vi "fpga_test.vi"() -> ()   [LabVIEW 2012]
uses:
  <vilib>/Utility/file.llb/Read From Spreadsheet File (I64).vi
panel:
  out "Array":i16[](array[numeric])
  out "unsigned 8bit integer":u8
  out "decimal integer string":string
  out "all rows 2":i64[][](array[numeric])
  out "all rows":i64[][](array[numeric])
  out "Starting address":u32
  out "State":enum16{"Wait for Command", "Read Buffer"}(ring)
  out "Is trigger?":bool
  out "count":u32
  out "Data":i16
  out "Timestamp":u64
  out "Channel":u8
  out "Trigger index":u32
  in  "Record Size only data":u32=95
  in  "circular buffer length":u32=1000
  in  "location":i16(ring) items=["Purdue", "NIKHEF", "Zurich", "???"]
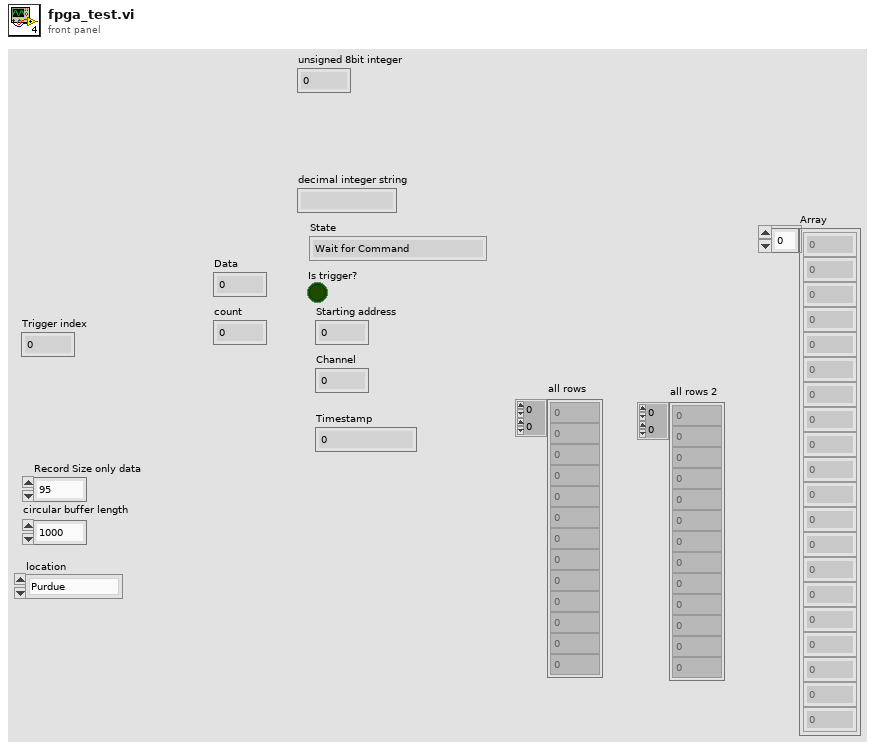
[diagram p1: front panel]
types:
  T1 = enum16{"open", "replace", "create", "open or create", "replace or create", "replace or create with confirmation"}
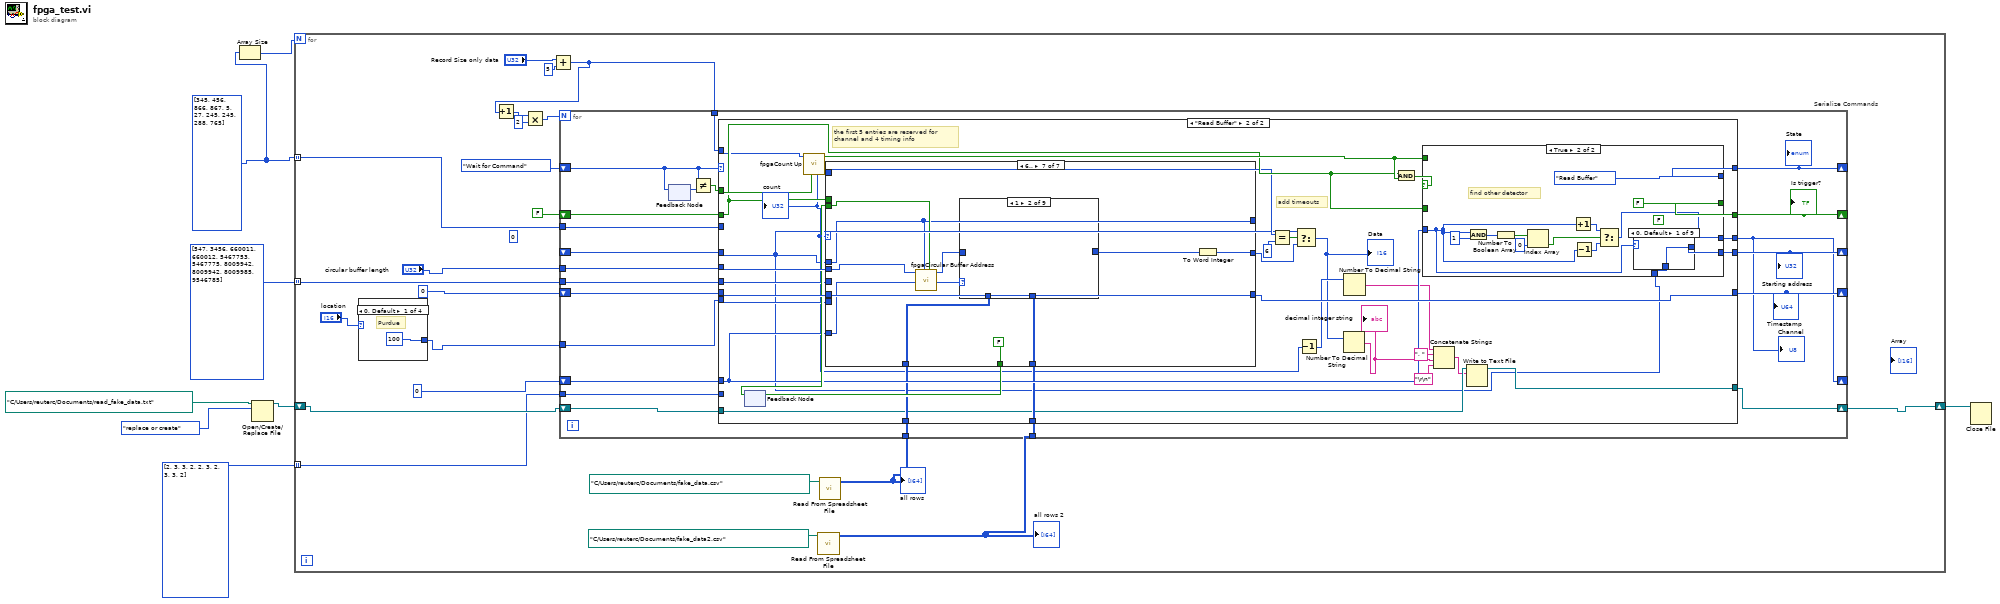
[diagram p0: block diagram]
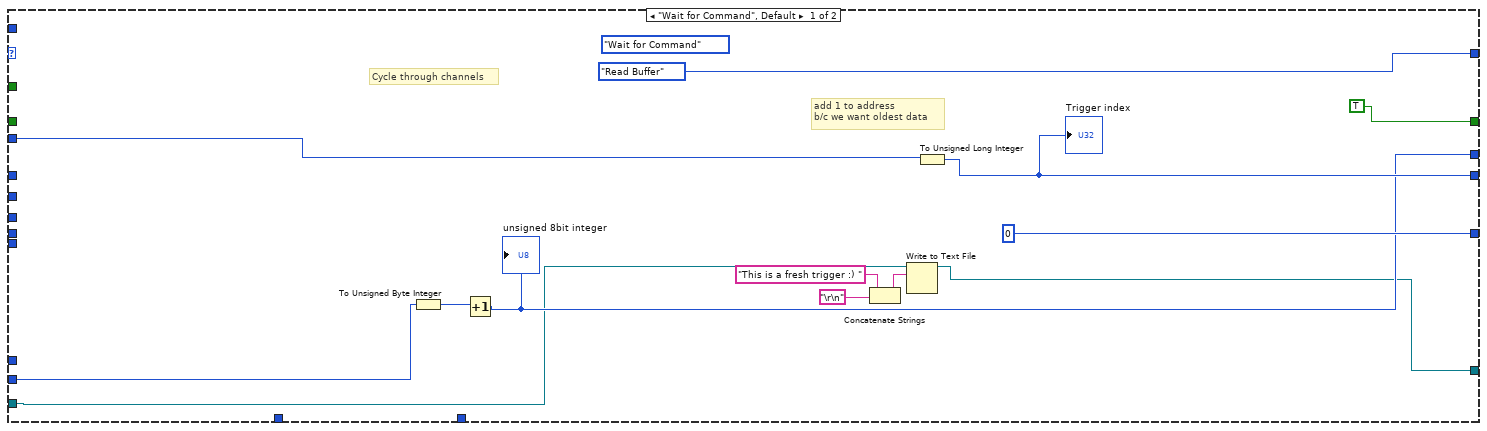
[diagram p2: hidden frame]
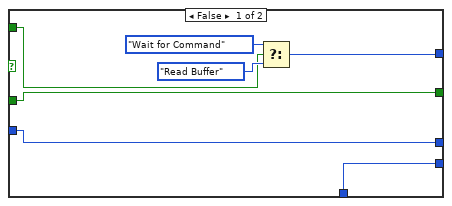
[diagram p3: hidden frame]
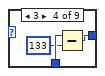
[diagram p6: hidden frame]
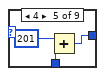
[diagram p7: hidden frame]
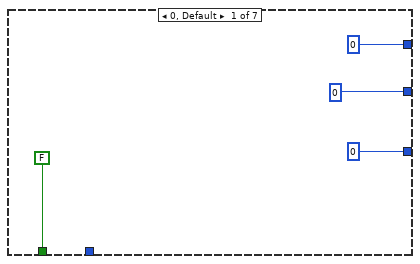
[diagram p12: hidden frame]
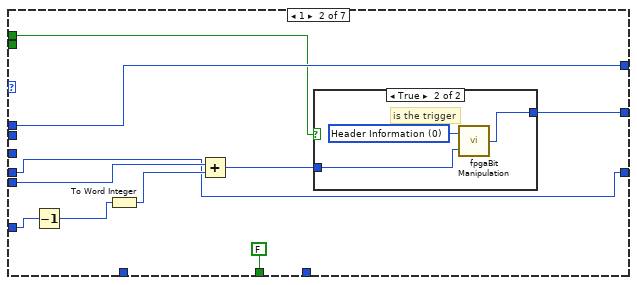
[diagram p13: hidden frame]
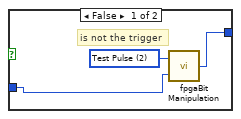
[diagram p14: hidden frame]
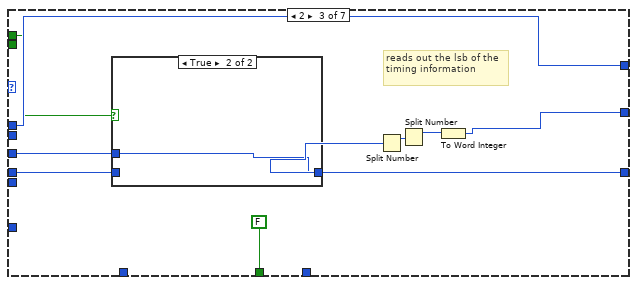
[diagram p15: hidden frame]
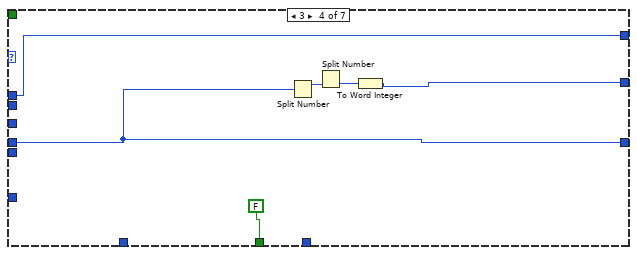
[diagram p17: hidden frame]
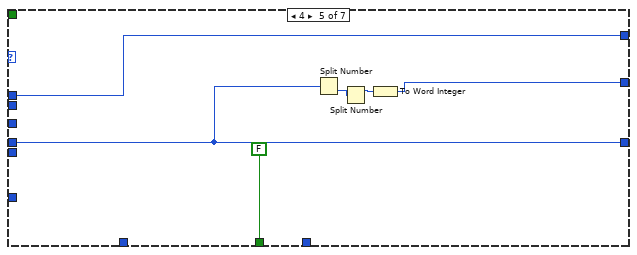
[diagram p18: hidden frame]
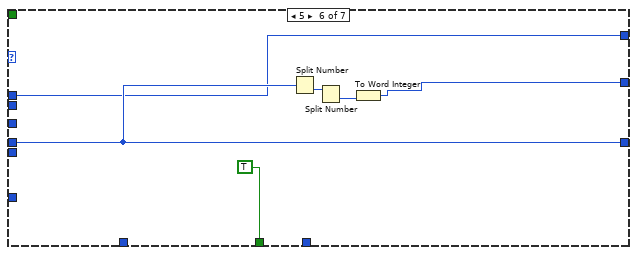
[diagram p19: hidden frame]
diagram:
  w4 = i32[] [345, 456, 866, 867, 5, 27, 245, 245, 288, 765]
  n1 = Array Size(array=w4) -> (size(s)=w3:i32)
  n2 = Open/Create/Replace File(file path (use dialog)=path "C:/Users/reuterc/Documents/read_fake_data.txt" ("file path (dialog if empty)"), operation (0:open)=T1."replace or create") -> (refnum out=w5:refnum<file>)  [unwired: 4 in, 2 out]
  n3 = for {
    N: w3 -> [_]
    shift-right: [w13] -> w8
    shift-left: w5 -> [w12]
    tunnel: w4 -> [w11] mode=indexing
    tunnel: i32[] [2, 3, 3, 2, 2, 3, 2, 3, 3, 2] -> [w10] mode=indexing
    tunnel: u64[] [547, 3456, 660011, 660012, 5467753, 5467775, 8009942, 8009942, 8009985, 9546785] -> [w9] mode=indexing
    (unwired) 0 ("element")
    n4 = case shown="0, Default" "location" {
      tunnel: [i16 100 i16 200 i16 300 i16 400] -> w29
      frame 0, Default {
        # "Purdue"
      }
      frame 1 {
        # "NIKHEF"
      }
      frame 2 {
        # "Zurich"
      }
      frame 3 {
        # "???"
      }
    }
    n5 = Add(x="Record Size only data", y=u32 5) -> (x+y=w17:u32)
    n6 = Increment(x=w17) -> (x+1=w16:u32)
    n7 = Multiply(x=w16, y=u32 2) -> (x*y=w14:u32)
    n8 = call-poly <vilib>:"Read From Spreadsheet File.vi"("file path (dialog if empty)"=path "C:/Users/reuterc/Documents/fake_data2.csv") -> ("all rows"=w22:i64[][])  [unwired: 6 in, 4 out]
    "all rows 2" <- w22
    n9 = call-poly <vilib>:"Read From Spreadsheet File.vi"("file path (dialog if empty)"=path "C:/Users/reuterc/Documents/fake_data.csv") -> ("all rows"=w23:i64[][])  [unwired: 6 in, 4 out]
    "all rows" <- w23
    n10 = for "Serialize Commands" {
      N: w14 -> [_]
      shift-right: [w49] -> _
      shift-left: enum16{"Wait for Command", "Read Buffer"}."Wait for Command" -> [w47]
      shift-right: [w52] -> _
      shift-left: _ -> [w51]
      shift-right: [w34] -> _
      shift-left: u8 0 ("t") -> [w50]
      shift-right: [w45] -> _
      shift-left: u64 0 ("Element") -> [w44]
      shift-right: [w42] -> _
      shift-left: FALSE -> [w43]
      tunnel: w29 -> [w41]
      tunnel: "circular buffer length" -> [w40]
      tunnel: w23 -> [w39]
      tunnel: w22 -> [w38]
      tunnel: w17 -> [w37]
      shift-right: [w36] -> w13
      shift-left: w12 -> [w35]
      tunnel: w11 -> [w33]
      tunnel: w10 -> [w32]
      tunnel: w9 -> [w31]
      n11 = feedback-in #1(w47) -> ()
      n12 = feedback #1() -> (w48:enum16{"Wait for Command", "Read Buffer"})  [unwired: 1 in]
      n13 = Not Equal?(x=w47, y=w48) -> (x != y?=w46:bool)
      n14 = case shown="\"Read Buffer\"" w47 {
        tunnel: w37 -> [_ w83]
        tunnel: w50 -> [_ w91]
        tunnel: [w63 w66] -> w52
        tunnel: w51 -> [_ w67]
        tunnel: [enum16{"Wait for Command", "Read Buffer"}."Read Buffer" w88] -> w49
        tunnel: w40 -> [_ w98]
        tunnel: w46 -> [_ w97]
        tunnel: [u64 0 ("Element") w96] -> w45
        tunnel: w44 -> [_ w95]
        tunnel: w41 -> [_ w92]
        tunnel: w43 -> [_ w86]
        tunnel: [TRUE w89] -> w42
        tunnel: w39 -> [_ w85]
        tunnel: w38 -> [_ w84]
        tunnel: [w60 w82] -> w34
        tunnel: [w58 w81] -> w36
        tunnel: w35 -> [w59 w80]
        tunnel: w33 -> [w54 _]
        tunnel: w32 -> [w53 _]
        tunnel: w31 -> [_ w73]
        frame "Wait for Command", Default {
          (unwired) enum16{"Wait for Command", "Read Buffer"}."Wait for Command"
          # "add 1 to address\nb/c we want oldest data"
          # "Cycle through channels"
          n15 = To Unsigned Byte Integer(number=w53) -> (unsigned 8bit integer=w61:u8)
          n16 = Increment(x=w61) -> (x+1=w60:u8)
          "unsigned 8bit integer" <- w60
          n17 = Concatenate Strings("This is a fresh trigger :) " ("text"), "\r\n") -> (w56:string)
          n18 = Write to Text File(file (use dialog)=w59, text=w56) -> (refnum out=w58:refnum<file>)  [unwired: 2 in, 2 out]
          n19 = To Unsigned Long Integer(number=w54) -> (unsigned 32bit integer=w63:u32)
          "Trigger index" <- w63
        }
        frame "Read Buffer" {
          # "the first 5 entries are reserved for channel and 4 timing info"
          # "add timeouts"
          n20 = feedback #2() -> (w94:bool)  [unwired: 1 in]
          n21 = call "fpgaCount Up.vi"("Reset?"=w97, "goal"=w83) -> ("Count Met"=w87:bool, "count"=w70:u32)  [unwired: 8 in]
          "count" <- w70
          n22 = case shown="6.." w70 {
            tunnel: w91 -> [_ w142 _ _ _ _ w186]
            tunnel: w67 -> [_ w145 w158 w165 w171 w177 w187]
            tunnel: w98 -> [_ _ _ _ _ _ w189]
            tunnel: [i16 0 ("Data") w143 w160 w163 w169 w176 w185] -> w69
            tunnel: w94 -> [_ _ _ _ _ _ w188]
            tunnel: [u64 0 ("Element") w136 w155 w166 w172 w178 w190] -> w96
            tunnel: w95 -> [_ w136 w154 w166 w172 w178 w190]
            tunnel: [u32 0 ("Element") w145 w158 w165 w171 w177 w187] -> _
            tunnel: [FALSE FALSE FALSE FALSE FALSE TRUE FALSE] -> w93
            tunnel: w92 -> [_ w138 _ _ _ _ _]
            tunnel: w86 -> [_ w137 w153 _ _ _ _]
            tunnel: w70 -> [_ _ _ _ _ _ _]
            tunnel: w85 -> [_ _ _ _ _ _ w183]
            tunnel: w84 -> [_ _ _ _ _ _ w181]
            tunnel: w73 -> [_ _ w152 _ _ _ _]
            frame 0, Default {
            }
            frame 1 {
              n23 = Decrement(x=w142) -> (x-1=w141:u8)
              n24 = To Word Integer(number=w141) -> (16bit integer=w140:i16)
              n25 = Add(x=w138, y=w140) -> (x+y=w139:i16)
              n26 = case shown="True" w137 {
                tunnel: [w146 w150] -> w143
                tunnel: w139 -> [w147 w149]
                frame False {
                  w148 = u16 2 items=["Header Information", "Particle Pulse", "Test Pulse"] ("Pulse Type")
                  # "is not the trigger"
                  n27 = call "fpgaBit Manipulation.vi"("Pulse Type"=w148, "Integer to be written"=w147) -> ("Integer Written"=w146:i16)  [unwired: 2 in]
                }
                frame True {
                  w151 = u16 0 items=["Header Information", "Particle Pulse", "Test Pulse"] ("Pulse Type")
                  # "is the trigger"
                  n28 = call "fpgaBit Manipulation.vi"("Pulse Type"=w151, "Integer to be written"=w149) -> ("Integer Written"=w150:i16)  [unwired: 2 in]
                }
              }
            }
            frame 2 {
              # "reads out the lsb of the timing information"
              n29 = case shown="True" w153 {
                tunnel: [w161 w162] -> w155
                tunnel: w154 -> [w161 _]
                tunnel: w152 -> [_ w162]
                frame False {
                }
                frame True {
                }
              }
              n30 = Split Number(x=w155) -> (hi(x)=w157:u32)  [unwired: 1 out]
              n31 = Split Number(x=w157) -> (hi(x)=w156:u16)  [unwired: 1 out]
              n32 = To Word Integer(number=w156) -> (16bit integer=w160:i16)
            }
            frame 3 {
              n33 = Split Number(x=w166) -> (hi(x)=w168:u32)  [unwired: 1 out]
              n34 = Split Number(x=w168) -> (lo(x)=w167:u16)  [unwired: 1 out]
              n35 = To Word Integer(number=w167) -> (16bit integer=w163:i16)
            }
            frame 4 {
              n36 = Split Number(x=w172) -> (lo(x)=w174:u32)  [unwired: 1 out]
              n37 = Split Number(x=w174) -> (hi(x)=w173:u16)  [unwired: 1 out]
              n38 = To Word Integer(number=w173) -> (16bit integer=w169:i16)
            }
            frame 5 {
              n39 = Split Number(x=w178) -> (lo(x)=w180:u32)  [unwired: 1 out]
              n40 = Split Number(x=w180) -> (lo(x)=w179:u16)  [unwired: 1 out]
              n41 = To Word Integer(number=w179) -> (16bit integer=w176:i16)
            }
            frame 6.. {
              n42 = call "fpgaCircular Buffer Address.vi"("Reset?"=w188, "Starting Address"=w187, "circular buffer length"=w189) -> ("Address"=w184:u32)  [unwired: 8 in]
              n43 = case shown="1" w186 {
                tunnel: w184 -> [_ _ _ w194 w198 _ _ _ _]
                tunnel: w183 -> [_ _ _ w195 _ _ _ _ _]
                tunnel: [_ _ _ w193 w196 _ _ _ _] -> w182
                tunnel: w181 -> [_ _ _ _ w199 _ _ _ _]
                frame Default {
                  # "Error"
                }
                frame 1 {
                }
                frame 2 {
                }
                frame 3 {
                  n44 = Index Array(array=w195, index (row)=w194, index (col)=0 ("disabled index (col)")) -> (element=w193:i64)
                }
                frame 4 {
                  n45 = Index Array(array=w199, index (row)=w198, index (col)=0 ("disabled index (col)")) -> (element=w196:i64)
                }
                frame 5 {
                }
                frame 6 {
                }
                frame 7 {
                }
                frame 8 {
                }
              }
              n46 = To Word Integer(number=w182) -> (16bit integer=w185:i16)
            }
          }
          n47 = feedback-in #2(w93) -> ()
          n48 = Equal?(x=w70, y=u32 6 ("f")) -> (x = y?=w72:bool)
          n49 = Select(t=w67, s=w72, f=w69) -> (s? t:f=w68:u32)
          "Data" <- w68
          n50 = Decrement(x=w70) -> (x-1=w74:u32)
          n51 = Number To Decimal String(number=w68) -> (decimal integer string=w78:string)  [unwired: 1 in]
          "decimal integer string" <- w78
          n52 = Number To Decimal String(number=w74) -> (decimal integer string=w76:string)  [unwired: 1 in]
          n53 = And(x=w86, y=w87) -> (x .and. y?=w90:bool)
          n54 = case shown="True" w90 {
            tunnel: w91 -> [w105 w106]
            tunnel: [w105 w107] -> w82
            tunnel: [w104 FALSE] -> w89
            tunnel: w86 -> [w104 _]
            tunnel: [w101 enum16{"Wait for Command", "Read Buffer"}."Read Buffer"] -> w88
            tunnel: w87 -> [w100 _]
            tunnel: w67 -> [w99 w109]
            tunnel: [w99 w108] -> w66
            frame False {
              n55 = Select(t=enum16{"Wait for Command", "Read Buffer"}."Wait for Command", s=w100, f=enum16{"Wait for Command", "Read Buffer"}."Read Buffer") -> (s? t:f=w101:enum16{"Wait for Command", "Read Buffer"})
            }
            frame True {
              (unwired) FALSE
              # "find other detector"
              n56 = And(x=w106, y=u8 1) -> (x .and. y?=w113:u8)
              n57 = Number To Boolean Array(number=w113) -> (Boolean array=w112:bool[])
              n58 = Index Array(array=w112, index=0) -> (element=w110:bool)
              n59 = Increment(x=w106) -> (x+1=w116:u8)
              n60 = Decrement(x=w106) -> (x-1=w115:u8)
              n61 = Select(t=w116, s=w110, f=w115) -> (s? t:f=w107:u8)
              n62 = case shown="0, Default" w106 {
                tunnel: [w119 w120 w121 w122 w125 w128 w129 w130 w131] -> w108
                tunnel: w109 -> [w119 w120 w121 w124 w127 w128 w129 w130 w131]
                frame 0, Default {
                }
                frame 1 {
                }
                frame 2 {
                }
                frame 3 {
                  n63 = Subtract(x=w124, y=u32 133) -> (x-y=w122:u32)
                }
                frame 4 {
                  n64 = Add(x=u32 201, y=w127) -> (x+y=w125:u32)
                }
                frame 5 {
                }
                frame 6 {
                }
                frame 7 {
                }
                frame 8 {
                }
              }
            }
          }
          n65 = Concatenate Strings(w76, ", " ("string"), w78, "\r\n") -> (w79:string)
          n66 = Write to Text File(file (use dialog)=w80, text=w79) -> (refnum out=w81:refnum<file>)  [unwired: 2 in, 2 out]
        }
      }
      "Channel" <- w34
      "Timestamp" <- w45
      "Is trigger?" <- w42
      "State" <- w49
      "Starting address" <- w52
    }
  }
  n67 = Close File(refnum=w8) -> ()  [unwired: 1 in, 2 out]
